vi "Read TTB record.vi"(8 "error in":errorcluster, 11 "Refnum":refnum<file>) -> (0 "error out":errorcluster, 1 "milliseconds":u16, 2 "seconds":u32, 3 "Duplicate Refnum":refnum<file>)   [LabVIEW 2016]
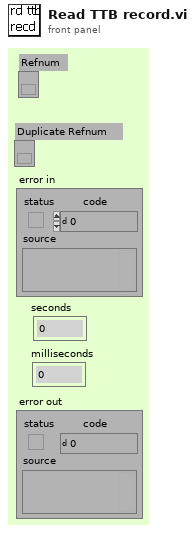
[diagram p1: front panel]
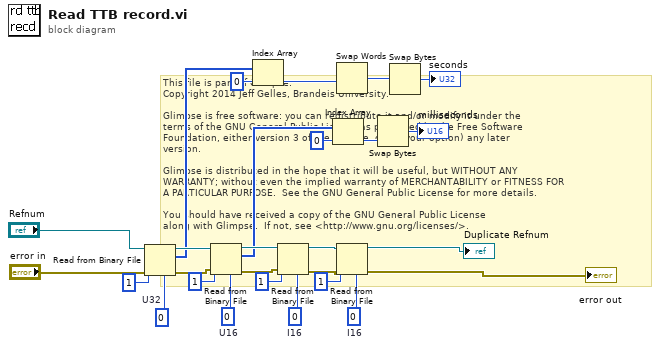
[diagram p0: block diagram]
diagram:
  w19 = i16 0  # I16
  w22 = i16 0  # I16
  w23 = u16 0  # U16
  w27 = u32 0  # U32
  # "This file is part of Glimpse. \nCopyright 2014 Jeff Gelles, Brandeis University.    \n\nGlimpse is free software: you can redistribute it and/or modify it under the \nterms of the GNU General Public License as published by the Free Software \nFoundation, either version 3 of the License, or (at your option) any later \nversion.\n\nGlimpse is distributed in the hope that it will be useful, but WITHOUT ANY \nWARRANTY; without even the implied warranty of MERCHANTABILITY or FITNESS FOR \nA PARTICULAR PURPOSE.  See the GNU General Public License for more details.\n\nYou should have received a copy of the GNU General Public License\nalong with Glimpse.  If not, see <http://www.gnu.org/licenses/>."
  n1 = Read from Binary File(5:w27, 8:"error in", 10:1 ("count"), 11:"Refnum") -> (0:w18:errorcluster, 2:w12:u32[], 3:w15:refnum<file>)  [unwired: 3 out]
  n2 = Read from Binary File(5:w23, 8:w18, 10:1 ("count"), 11:w15) -> (0:w17:errorcluster, 2:w10:u16[], 3:w14:refnum<file>)  [unwired: 3 out]
  n3 = Index Array(array=w12, index=0) -> (element=w4:u32)
  n4 = Read from Binary File(5:w22, 8:w17, 10:1 ("count"), 11:w14) -> (0:w16:errorcluster, 3:w13:refnum<file>)  [unwired: 4 out]
  n5 = Index Array(array=w10, index=0) -> (element=w2:u16)
  n6 = Swap Words(1:w4) -> (0:w11:u32)
  n7 = Read from Binary File(5:w19, 8:w16, 10:1 ("count"), 11:w13) -> (0:→"error out":errorcluster, 3:→"Duplicate Refnum":refnum<file>)  [unwired: 4 out]
  n8 = Swap Bytes(anything=w2) -> (byte swapped=→"milliseconds":u16)
  n9 = Swap Bytes(anything=w11) -> (byte swapped=→"seconds":u32)
